vi "1Dinterp.vi"() -> ()   [LabVIEW 2016]
uses:
  <vilib>/Math Plots/3D Math Plots/3D Surface/3D Surface XCtrl/3D Surface.xctl
  <vilib>/Math Plots/3D Math Plots/3D Surface/3D Surface Datatype/Public/Plot Helper (Matrix).vi
  <vilib>/Math Plots/3D Math Plots/3D Surface/3D Surface Datatype/3D Surface Datatype.lvclass
  <vilib>/measure/NI_MABase.lvlib
  <vilib>/gmath/NI_Gmath.lvlib
panel:
  in  "interp":i32=10
  out "XY Graph":cluster{"yi":dbl[], "xi used":dbl[]}(graph)
  out "dt":dbl
  in  "sampling info":cluster{"Fs":dbl, "#s":dbl}={"Fs"=4.0, "#s"=2.0}
  out "Waveform Graph":waveform(dbl)(graph)
  out "3D Surface":refnum<class "3D Plot Datatype.lvclass">[](xcontrol)
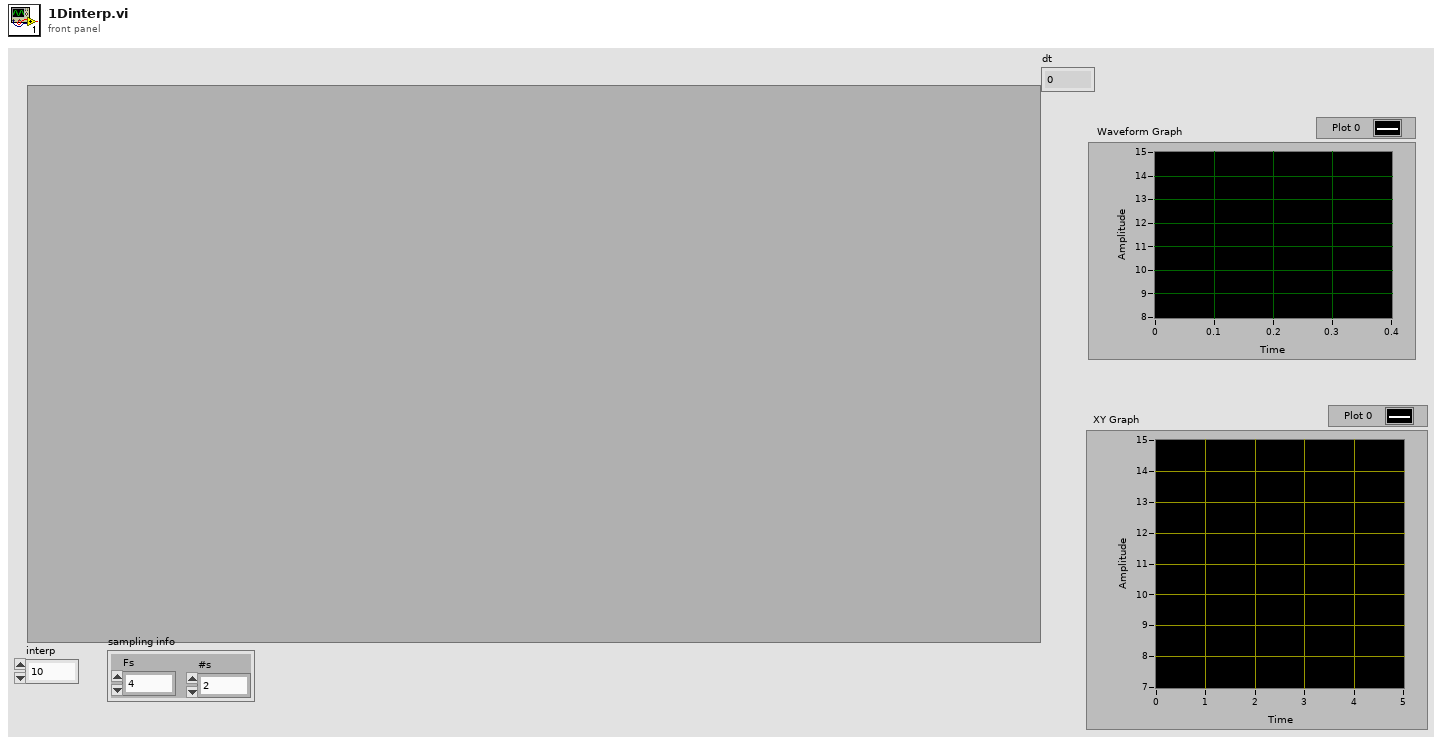
[diagram p1: front panel]
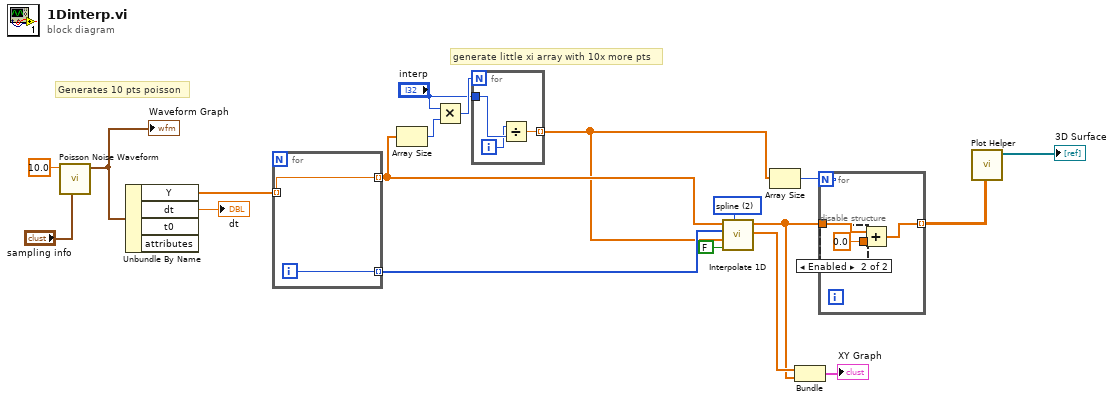
[diagram p0: block diagram]
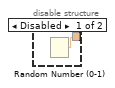
[diagram p2: hidden frame]
diagram:
  w8 = 2 items=["nearest", "linear", "spline", "cubic Hermite", "Lagrange"] ("method")
  # "generate little xi array with 10x more pts"
  # "Generates 10 pts poisson"
  n1 = call <vilib>:"Poisson Noise Waveform.vi"("sampling info"="sampling info", "mean"=10.0) -> ("signal out"=w17:waveform(dbl))  [unwired: 8 in, 1 out]
  "Waveform Graph" <- w17
  n2 = Unbundle By Name(w17) -> ("Y"=w15:dbl[], "dt"=→"dt":dbl)  [unwired: 2 out]
  n3 = for {
    tunnel: w15 -> [w21] mode=indexing
    tunnel: [w21] -> w5 mode=indexing
    tunnel: [w20] -> w13 mode=indexing
    i -> [w20]
  }
  n4 = Array Size(array=w5) -> (size(s)=w12:i32)
  n5 = Multiply(x="interp", y=w12) -> (x*y=w11:i32)
  n6 = for {
    N: w11 -> [_]
    tunnel: "interp" -> [w24]
    tunnel: [w22] -> w3 mode=indexing
    i -> [w23]
    n7 = Divide(x=w23, y=w24) -> (x/y=w22:dbl)
  }
  n8 = call <vilib>:"Interpolate 1D.vi"("method"=w8, "X is monotonic"=FALSE, "xi"=w3, "X"=w13, "Y"=w5) -> ("xi used"=w7:dbl[], "yi"=w2:dbl[])  [unwired: 4 in, 1 out]
  n9 = Array Size(array=w3) -> (size(s)=w4:i32)
  n10 = Bundle("xi used"=w7, "yi"=w2) -> (→"XY Graph":cluster{"xi used":dbl[], "yi":dbl[]})  [unwired: 1 in]
  n11 = for {
    N: w4 -> [_]
    tunnel: w2 -> [w26]
    tunnel: [w25] -> w1 mode=indexing
    n12 = disable-structure shown="Enabled" {
      disable-tunnel: [w28 0.0 ("number: 0 to 1")] -> w27
      frame Disabled {
        n13 = Random Number (0-1)() -> (number: 0 to 1=w28:dbl)
      }
      frame Enabled {
      }
    }
    n14 = Add(x=w26, y=w27) -> (x+y=w25:dbl[])
  }
  n15 = call-poly <vilib>:"Plot Helper.vi"("z matrix"=w1) -> ("3D Plot lvclass Array out"=→"3D Surface":refnum<class "3D Plot Datatype.lvclass">[])  [unwired: 5 in, 5 out]
